vi "AB_Engine_Update_Palette_Files.vi"(8 "error in":errorcluster, 9 "new paths":path[](array[path]), 10 "old paths":path[](array[path]), 11 "application reference":refnum<vi>) -> (0 "error out":errorcluster)   [LabVIEW 2020]
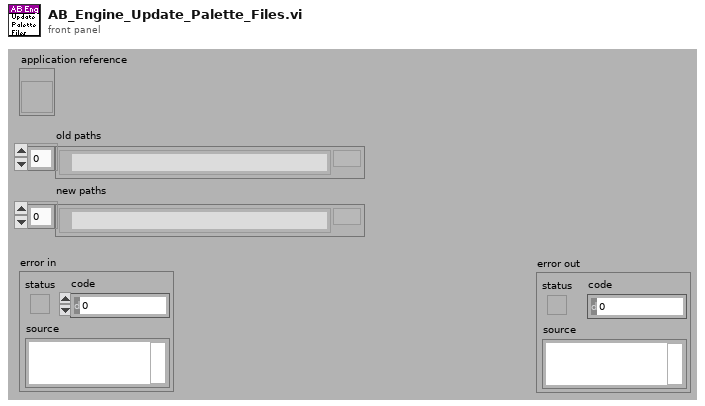
[diagram p1: front panel]
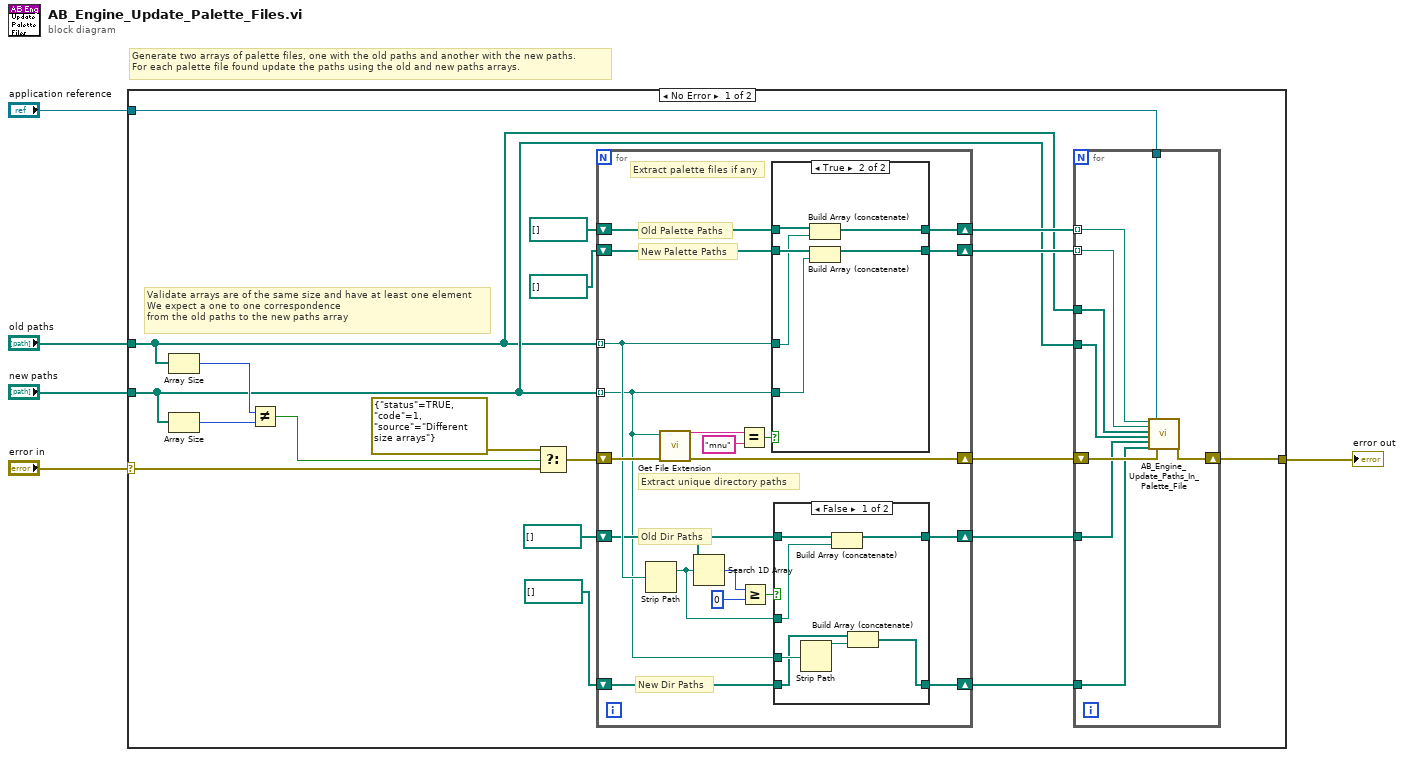
[diagram p0: block diagram]
diagram:
  # "Generate two arrays of palette files, one with the old paths and another with the new paths.\nFor each palette file found update the paths using the old and new paths arrays."
  n1 = case shown="No Error" "error in" {
    selector: "error in" -> [w15 w70]
    tunnel: [w19 w70] -> w1
    tunnel: "new paths" -> [w11 _]
    tunnel: "old paths" -> [w10 _]
    tunnel: "application reference" -> [w18 _]
    frame No Error {
      # "Validate arrays are of the same size and have at least one element\nWe expect a one to one correspondence \nfrom the old paths to the new paths array"
      n2 = Array Size(array=w10) -> (size(s)=w17:i32)
      n3 = Array Size(array=w11) -> (size(s)=w16:i32)
      n4 = Not Equal?(x=w17, y=w16) -> (x != y?=w12:bool)
      n5 = Select(t=errorcluster {"status"=TRUE, "code"=1, "source"="Different size arrays"}, s=w12, f=w15) -> (s? t:f=w14:errorcluster)
      n6 = for {
        tunnel: w11 -> [w34] mode=indexing
        tunnel: w10 -> [w41] mode=indexing
        shift-right: [w45] -> w21
        shift-left: path[] [] -> [w48]
        shift-right: [w46] -> w22
        shift-left: path[] [] -> [w47]
        shift-right: [w44] -> w20
        shift-left: w14 -> [w50]
        shift-right: [w39] -> w7
        shift-left: path[] [] -> [w36]
        shift-right: [w37] -> w6
        shift-left: path[] [] -> [w38]
        # "New Dir Paths"
        # "Old Dir Paths"
        # "Extract unique directory paths"
        # "New Palette Paths"
        # "Old Palette Paths"
        # "Extract palette files if any"
        n7 = Strip Path(path=w41) -> (stripped path=w35:path)  [unwired: 1 out]
        n8 = call <vilib>:"Get File Extension.vi"("error in (no error)"=w50, "file"=w34) -> ("error out"=w44:errorcluster, "lowercase file extension"=w52:string)  [unwired: 5 in, 3 out]
        n9 = Search 1D Array(1D array=w36, element=w35) -> (index of element=w42:i32)  [unwired: 1 in]
        n10 = Equal?(x=w52, y="mnu") -> (x = y?=w49:bool)
        n11 = Greater Or Equal?(x=w42, y=0) -> (x >= y?=w40:bool)
        n12 = case shown="True" w49 {
          tunnel: w34 -> [_ w64]
          tunnel: w41 -> [_ w65]
          tunnel: w48 -> [w63 w67]
          tunnel: w47 -> [w62 w69]
          tunnel: [w63 w66] -> w45
          tunnel: [w62 w68] -> w46
          frame False {
          }
          frame True {
            n13 = Build Array (concatenate)(w69, w65) -> (w68:path[])
            n14 = Build Array (concatenate)(w67, w64) -> (w66:path[])
          }
        }
        n15 = case shown="False" w40 {
          tunnel: w36 -> [w58 w61]
          tunnel: [w56 w61] -> w39
          tunnel: w38 -> [w54 w60]
          tunnel: [w53 w60] -> w37
          tunnel: w35 -> [w57 _]
          tunnel: w34 -> [w55 _]
          frame False {
            n16 = Strip Path(path=w55) -> (stripped path=w59:path)  [unwired: 1 out]
            n17 = Build Array (concatenate)(w58, w57) -> (w56:path[])
            n18 = Build Array (concatenate)(w54, w59) -> (w53:path[])
          }
          frame True {
          }
        }
      }
      n19 = for {
        tunnel: w22 -> [w26] mode=indexing
        tunnel: w21 -> [w27] mode=indexing
        shift-right: [w32] -> w19
        shift-left: w20 -> [w33]
        tunnel: w18 -> [w25]
        tunnel: w10 -> [w28]
        tunnel: w11 -> [w29]
        tunnel: w7 -> [w30]
        tunnel: w6 -> [w31]
        n20 = call <vilib>:"AB_Engine_Update_Paths_In_Palette_File.vi"("old palette path"=w26, "new palette path"=w27, "old paths"=w28, "new paths"=w29, "old dir paths"=w30, "new dir paths"=w31, "application reference"=w25, "error in"=w33) -> ("error out"=w32:errorcluster)  [unwired: 11 in]
      }
    }
    frame Error {
    }
  }
  "error out" <- w1
